vi "test Check If Custom Device Is Enabled.vi"(8 "error in":errorcluster, 11 "TestCase in":refnum<class "Scripting.lvclass">) -> (0 "error out":errorcluster, 3 "TestCase out":refnum<class "Scripting.lvclass">)   [LabVIEW 2020, in "Scripting.lvclass"]
uses:
  Scripting.lvclass
  <vilib>/addons/_JKI Toolkits/VI Tester/TestCase.llb/TestCase.lvclass
  Scripting/AIM MIL-STD-1553 Scripting.lvlib
  C:/dev/git/niveristand-custom-device-testing-tools/VeriStandScriptingTestCase/VeriStandScriptingTestCase.lvclass
  C:/Program Files (x86)/National Instruments/LabVIEW 2020/vi.lib/addons/_JKI Toolkits/VI Tester/TestCase.llb/TestCase.lvclass
  C:/dev/git/niveristand-aim-milStd1553-custom-device/Source/Custom Device Support/Tests/Unit/Scripting/Scripting.lvclass
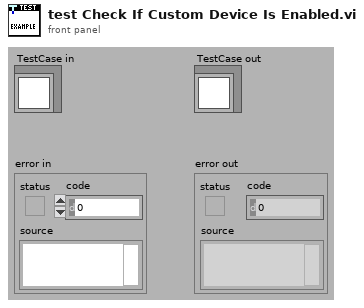
[diagram p1: front panel]
types:
  T1 = typedef "Custom Device API.lvlib/Custom Device Item Ref.ctl" = u64
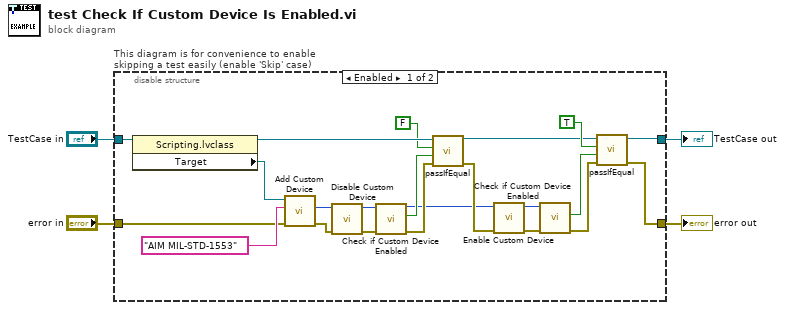
[diagram p0: block diagram]
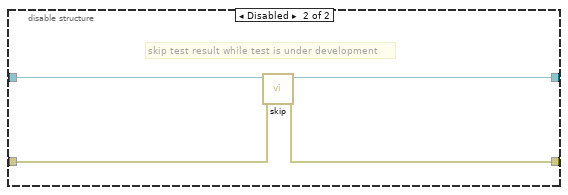
[diagram p2: hidden frame]
diagram:
  n1 = disable-structure "This diagram is for convenience to enable skipping a test easily (enable 'Skip' case)" shown="Enabled" {
    disable-tunnel: "TestCase in" -> [w25 w30]
    disable-tunnel: [w10 w28] -> w1
    disable-tunnel: [w11 w29] -> w3
    disable-tunnel: "error in" -> [w23 w27]
    frame Enabled {
      n2 = property class="Scripting.lvclass"(reference=w25) -> (reference out=w22:refnum<class "Scripting.lvclass">, "Target"=w24:refnum<k24>)  [unwired: 1 in, 1 out]
      n3 = call "Add Custom Device.vi"("error in"=w23, "custom device name"="AIM MIL-STD-1553" ("name"), "target"=w24) -> ("error out"=w21:errorcluster, "custom device"=w20:T1)  [unwired: 6 in, 1 out]
      n4 = call "Disable Custom Device.vi"("error in"=w21, "custom device ref"=w20) -> ("error out"=w18:errorcluster, "custom device ref out"=w19:T1)  [unwired: 8 in]
      n5 = call "Check if Custom Device Enabled.vi"("error in"=w18, "custom device ref"=w19) -> ("error out"=w17:errorcluster, "is enabled?"=w16:bool, "custom device ref out"=w5:T1)  [unwired: 7 in]
      n6 = call-dynamic "passIfEqual.vi"("error in (no error)"=w17, "y"=w16, "x"=FALSE ("is enabled?"), "TestCase in"=w22) -> ("error out"=w6:errorcluster, "TestCase out"=w9:refnum<class "Scripting.lvclass">)  [unwired: 6 in]
      n7 = call "Enable Custom Device.vi"("error in"=w6, "custom device ref"=w5) -> ("error out"=w7:errorcluster, "custom device ref out"=w8:T1)  [unwired: 8 in]
      n8 = call "Check if Custom Device Enabled.vi"("error in"=w7, "custom device ref"=w8) -> ("error out"=w12:errorcluster, "is enabled?"=w13:bool)  [unwired: 7 in, 1 out]
      n9 = call-dynamic "passIfEqual.vi"("error in (no error)"=w12, "y"=w13, "x"=TRUE ("is enabled?"), "TestCase in"=w9) -> ("error out"=w11:errorcluster, "TestCase out"=w10:refnum<class "Scripting.lvclass">)  [unwired: 6 in]
    }
    frame Disabled {
      # "skip test result while test is under development"
      n10 = call <vilib>:"skip.vi"("error in (no error)"=w27, "TestCase in"=w30) -> ("error out"=w29:errorcluster, "TestCase out"=w28:refnum<class "Scripting.lvclass">)  [unwired: 8 in]
    }
  }
  "error out" <- w3
  "TestCase out" <- w1
